vi "CheckBottom.vi"(0 "Chessboard":T2, 5 "ItemIndex":T1, 7 "StoneColor":u16, 11 "error in (no error)":errorcluster) -> (15 "error out":errorcluster)   [LabVIEW 2009]
uses:
  Controls/Chess.ctl
  Controls/ItemIndex.ctl
  BottomHaveSameStone.vi
  Controls/directions.ctl
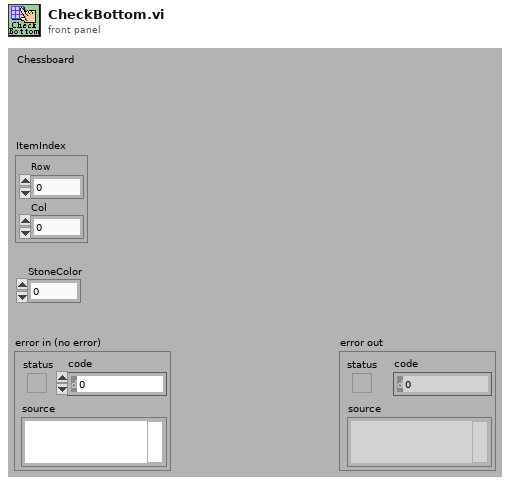
[diagram p1: front panel]
types:
  T1 = typedef "ItemIndex.ctl" = cluster{"Row":i32, "Col":i32}
  T2 = typedef "Chess.ctl" = u16[][]
  T3 = typedef "directions.ctl" = enum16{"Left", "Right", "Top", "Bottom", "TopLeft", "TopRight", "BottomLeft", "BottomRight", "ClearAll", "ReadAll"}
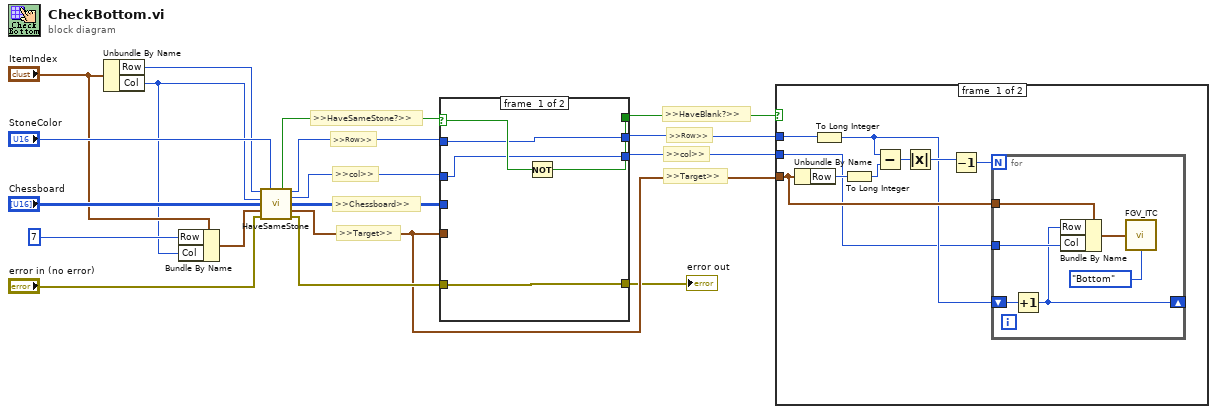
[diagram p0: block diagram]
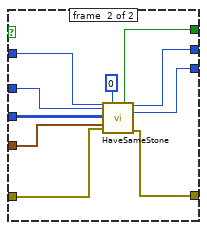
[diagram p3: hidden frame]
diagram:
  # ">>HaveBlank?>>"
  # ">>HaveSameStone?>>"
  # ">>Target>>"
  # ">>col>>"
  # ">>Row>>"
  # ">>Target>>"
  # ">>Chessboard>>"
  # ">>col>>"
  # ">>Row>>"
  n1 = Unbundle By Name("ItemIndex") -> ("Row"=w14:i32, "Col"=w1:i32)
  n2 = Bundle By Name(cluster="ItemIndex", "Row"=u32 7 ("Col"), "Col"=w1) -> (w13:T1)
  n3 = call-poly "HaveSameStone.vi"("Row in"=w14, "StoneColor"="StoneColor", "Col in"=w1, "Chessboard"="Chessboard", "TatgetIndex"=w13, "error in (no error)"="error in (no error)") -> ("HaveSameStone?"=w11:bool, "Row out"=w9:i32, "Col out"=w10:i32, "Chessboard out"=w12:T2, "SSIndex"=w4:T1, "error out"=w8:errorcluster)  [unwired: 4 in]
  n4 = case shown="True" w11 {
    selector: w11 -> [w23 _]
    tunnel: w4 -> [_ w32]
    tunnel: w12 -> [_ w31]
    tunnel: w10 -> [w19 w30]
    tunnel: w9 -> [w20 w29]
    tunnel: w8 -> [w21 w28]
    tunnel: [w22 w27] -> w7
    tunnel: [w21 w26] -> w3
    tunnel: [w20 w25] -> w6
    tunnel: [w19 w24] -> w5
    frame #0 {
      n5 = Not(x=w23) -> (.not. x?=w22:bool)
    }
    frame #1 {
      n6 = call-poly "HaveSameStone.vi"("Row in"=w29, "StoneColor"=u16 0, "Col in"=w30, "Chessboard"=w31, "TatgetIndex"=w32, "error in (no error)"=w28) -> ("HaveSameStone?"=w27:bool, "Row out"=w25:i32, "Col out"=w24:i32, "error out"=w26:errorcluster)  [unwired: 4 in, 2 out]
    }
  }
  "error out" <- w3
  n7 = case shown="False" w7 {
    tunnel: w6 -> [w36 _]
    tunnel: w5 -> [w34 _]
    tunnel: w4 -> [w42 _]
    frame #0 {
      n8 = Unbundle By Name(w42) -> ("Row"=w41:i32)
      n9 = To Long Integer(number=w36) -> (32bit integer=w35:i32)
      n10 = To Long Integer(number=w41) -> (32bit integer=w40:i32)
      n11 = Subtract(x=w35, y=w40) -> (x-y=w39:i32)
      n12 = Absolute Value(x=w39) -> (abs(x)=w37:i32)
      n13 = Decrement(x=w37) -> (x-1=w38:i32)
      n14 = for {
        N: w38 -> [_]
        shift-right: [w43] -> _
        shift-left: w35 -> [w48]
        tunnel: w42 -> [w47]
        tunnel: w34 -> [w44]
        n15 = Increment(x=w48) -> (x+1=w43:i32)
        n16 = Bundle By Name(cluster=w47, "Row"=w43, "Col"=w44) -> (w46:T1)
        n17 = call "FGV_ITC.vi"("ItemIndex"=w46, "Action"=directions."Bottom") -> ()  [unwired: 12 in, 2 out]
      }
    }
    frame #1 {
    }
  }
